vi "changing_directories.vi"() -> ()   [LabVIEW 2019]
panel:
  out "appended path 2":path
  out "appended path":path
  out "selected path":path
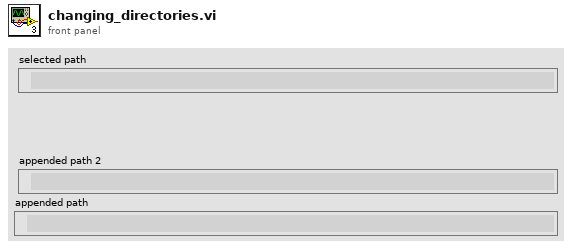
[diagram p1: front panel]
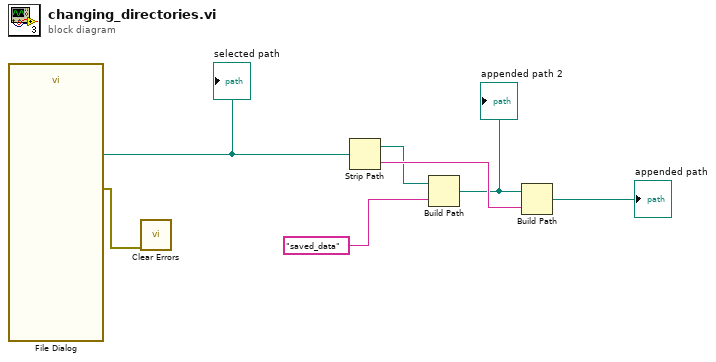
[diagram p0: block diagram]
diagram:
  n1 = call "File Dialog"() -> ("selected path"=w5:path, "error out"=w7:errorcluster)  [unwired: 12 in, 2 out]
  "selected path" <- w5
  n2 = call <vilib>:"Clear Errors.vi"("error in (no error)"=w7) -> ()  [unwired: 5 in, 2 out]
  n3 = Strip Path(path=w5) -> (stripped path=w1:path, name=w4:string)
  n4 = Build Path(base path=w1, name or relative path="saved_data") -> (appended path=w3:path)
  "appended path 2" <- w3
  n5 = Build Path(base path=w3, name or relative path=w4) -> (appended path=→"appended path":path)
